vi "cDAQ Create Cal File Array (RIO).vi"() -> (0 "Cal Target Array":string[](array[string]), 3 "Cal Log OUT":string[][](array[string]))   [LabVIEW 2013]
uses:
  Type Defs/Units Type Def (DAQ Rack).ctl
  Type Defs/cDAQ Type Def (cDAQ).ctl
panel:
  in  "Channel to Cal":T1
  in  "Cal Unit":T2
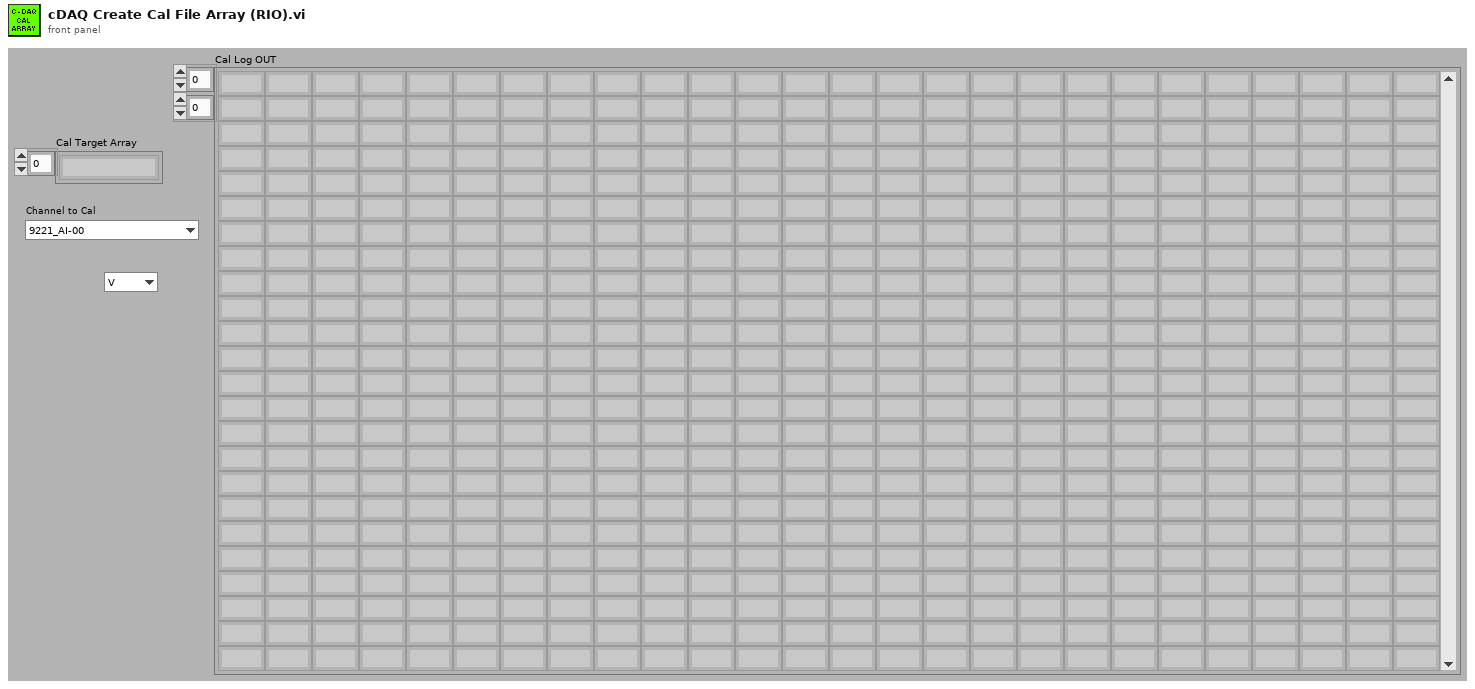
[diagram p1: front panel]
types:
  T1 = typedef "cDAQ Type Def (cDAQ).ctl" = enum16{"9221_AI-00", "9221_AI-01", "9221_AI-02", "9221_AI-03", "9221_AI-04", "9221_AI-05", "9221_AI-06", "9221_AI-07", "9205_AI-00", "9205_AI-01", "9205_AI-02", "9205_AI-03", "9205_AI-04", "9205_AI-05", "9205_AI-06", "9205_AI-07", "9208_AI-00", "9208_AI-01", "9208_AI-02", "9208_AI-03", "9208_AI-04", "9208_AI-05", "9208_AI-06", "9208_AI-07", "9211_TC-00", "9211_TC-01", "9211_TC-02", "9211_TC-03"}
  T2 = typedef "Units Type Def (DAQ Rack).ctl" = enum16{"V", "mA", "A", "Hz", "deg C"}
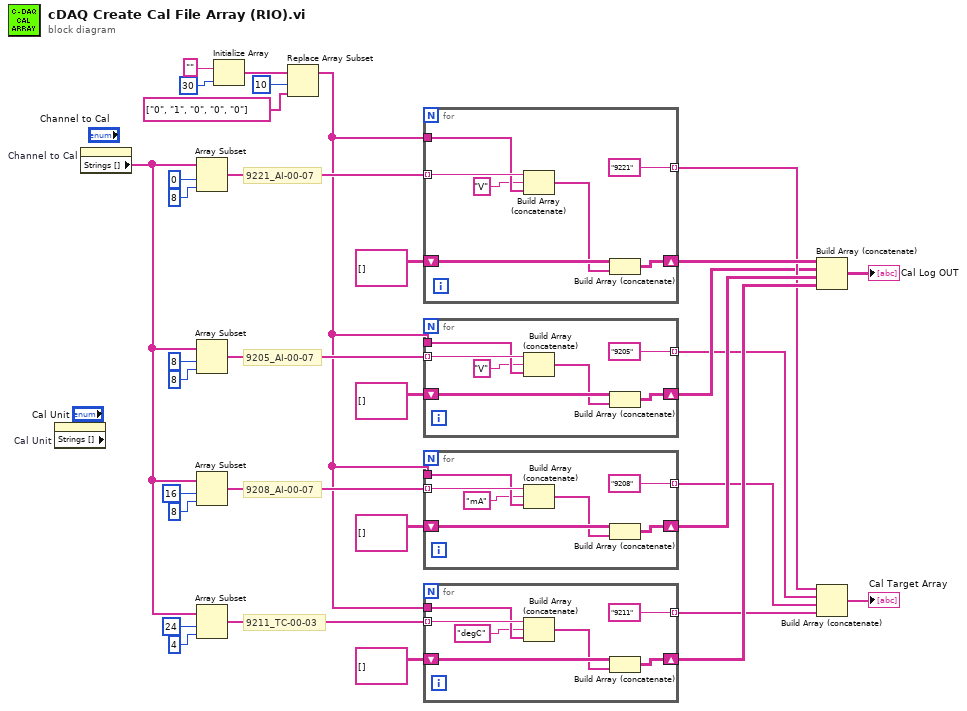
[diagram p0: block diagram]
diagram:
  # "9211_TC-00-03"
  # "9208_AI-00-07"
  # "9205_AI-00-07"
  # "9221_AI-00-07"
  n1 = property on="Cal Unit" class="Enum (strict)" props=["Strings []"]() -> ()  [unwired: 2 in, 3 out]
  n2 = property on="Channel to Cal" class="Enum (strict)"() -> ("Strings []"=w5:string[])  [unwired: 2 in, 2 out]
  n3 = Array Subset(array=w5, index=0, length=8) -> (w29:string[])
  n4 = Array Subset(array=w5, index=8, length=8) -> (w8:string[])
  n5 = Array Subset(array=w5, index=16, length=8) -> (w24:string[])
  n6 = Array Subset(array=w5, index=24, length=4) -> (w17:string[])
  n7 = Initialize Array("", 30 ("dimension size")) -> (w3:string[])
  n8 = Replace Array Subset(array=w3, new element=string[] ["0", "1", "0", "0", "0"], index=10) -> (w2:string[])
  n9 = for {
    tunnel: w29 -> [w40] mode=indexing
    tunnel: w2 -> [w39]
    shift-right: [w37] -> w23
    shift-left: string[][] [] ("Cal Log OUT") -> [w38]
    tunnel: ["9221"] -> w13 mode=indexing
    n10 = Build Array (concatenate)(w40, "V" ("element"), w39) -> (w36:string[])
    n11 = Build Array (concatenate)(w38, w36) -> (w37:string[][])
  }
  n12 = for {
    tunnel: w8 -> [w45] mode=indexing
    tunnel: w2 -> [w43]
    shift-right: [w46] -> w7
    shift-left: string[][] [] ("Cal Log OUT") -> [w47]
    tunnel: ["9205"] -> w6 mode=indexing
    n13 = Build Array (concatenate)(w45, "V" ("element"), w43) -> (w44:string[])
    n14 = Build Array (concatenate)(w47, w44) -> (w46:string[][])
  }
  n15 = for {
    tunnel: w24 -> [w52] mode=indexing
    tunnel: w2 -> [w50]
    shift-right: [w53] -> w21
    shift-left: string[][] [] ("Cal Log OUT") -> [w54]
    tunnel: ["9208"] -> w12 mode=indexing
    n16 = Build Array (concatenate)(w52, "mA" ("element"), w50) -> (w51:string[])
    n17 = Build Array (concatenate)(w54, w51) -> (w53:string[][])
  }
  n18 = for {
    tunnel: w17 -> [w59] mode=indexing
    tunnel: w2 -> [w57]
    shift-right: [w60] -> w16
    shift-left: string[][] [] ("Cal Log OUT") -> [w61]
    tunnel: ["9211"] -> w14 mode=indexing
    n19 = Build Array (concatenate)(w59, "degC" ("element"), w57) -> (w58:string[])
    n20 = Build Array (concatenate)(w61, w58) -> (w60:string[][])
  }
  n21 = Build Array (concatenate)(w23, w7, w21, w16) -> (→"Cal Log OUT":string[][])
  n22 = Build Array (concatenate)(w13, w6, w12, w14) -> (→"Cal Target Array":string[])
